vi "getParameters.vi"(11 "ExitMaintenanceCommand in":refnum<class "ExitMaintenanceCommand.lvclass">) -> (2 "Parameters":T1, 3 "ExitMaintenanceCommand out":refnum<class "ExitMaintenanceCommand.lvclass">)   [LabVIEW 2016, in "ExitMaintenanceCommand.lvclass"]
uses:
  ExitMaintenanceCommand.lvclass
  DataTypes/Topics/CommandExitMaintenance.ctl
  DataTypes/Topics/Parts/CommandId.ctl
  ExitMaintenanceCommand.lvclass/ExitMaintenanceCommand.ctl
  DataTypes/Topics/M1M3SupportTopics.lvlib
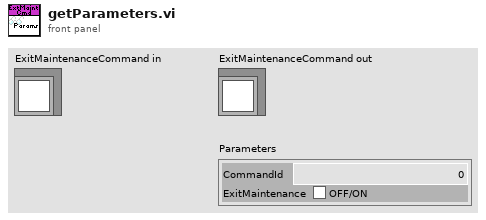
[diagram p1: front panel]
types:
  T1 = typedef "M1M3SupportTopics.lvlib/CommandExitMaintenance.ctl" = cluster{"CommandId":T2, "ExitMaintenance":bool}
  T2 = typedef "M1M3SupportTopics.lvlib/CommandId.ctl" = i32
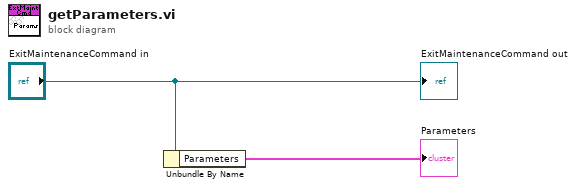
[diagram p0: block diagram]
diagram:
  n1 = Unbundle By Name("ExitMaintenanceCommand in") -> ("Parameters"=→"Parameters":T1)
  "ExitMaintenanceCommand out" <- "ExitMaintenanceCommand in"
